vi "Set Position Limits.vi"(8 "error in (no error)":errorcluster, 9 "min dist (m)":dbl, 10 "max dist (m)":dbl, 11 "KUKA youBot gripper motor in":refnum<class "NI_Robotics_KUKA youBot Gripper Motor.lvclass">) -> (0 "error out":errorcluster, 3 "KUKA youBot gripper motor out":refnum<class "NI_Robotics_KUKA youBot Gripper Motor.lvclass">)   [LabVIEW 2017, in "NI_Robotics_KUKA youBot Host.lvlib" / "NI_Robotics_KUKA youBot Gripper Motor.lvclass"]
uses:
  <vilib>/robotics/KUKA youBot/Motor/Gripper Motor/NI_Robotics_KUKA youBot Gripper Motor.lvclass
  <vilib>/robotics/KUKA youBot/Motor/Gripper Motor/NI_Robotics_KUKA youBot Gripper Motor.lvclass/NI_Robotics_KUKA youBot Gripper Motor.ctl
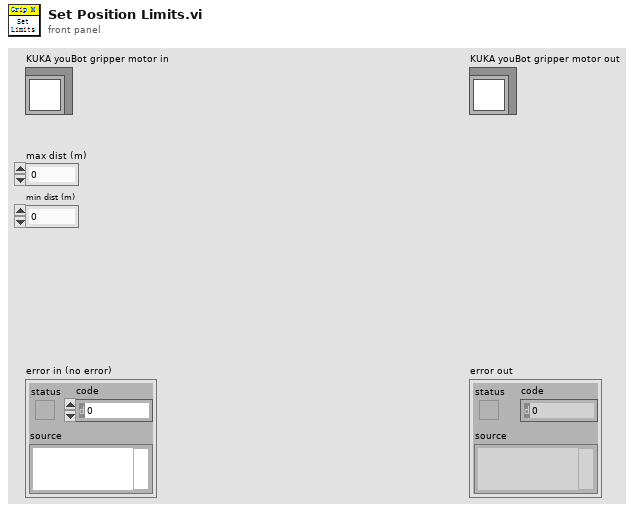
[diagram p1: front panel]
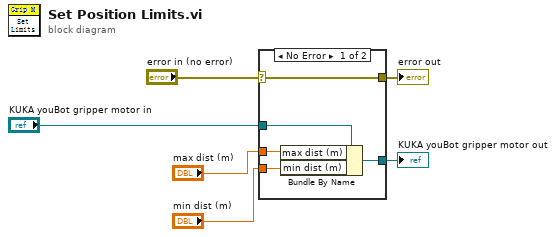
[diagram p0: block diagram]
diagram:
  n1 = case shown="No Error" "error in (no error)" {
    selector: "error in (no error)" -> [w11 w13]
    tunnel: [w11 w13] -> w5
    tunnel: [w7 w12] -> w3
    tunnel: "KUKA youBot gripper motor in" -> [w10 w12]
    tunnel: "max dist (m)" -> [w9 _]
    tunnel: "min dist (m)" -> [w8 _]
    frame No Error {
      n2 = Bundle By Name(cluster=w10, "max dist (m)"=w9, "min dist (m)"=w8) -> (w7:refnum<class "NI_Robotics_KUKA youBot Gripper Motor.lvclass">)
    }
    frame Error {
    }
  }
  "error out" <- w5
  "KUKA youBot gripper motor out" <- w3
